vi "LINX I2C Write Test App.vi"() -> ()   [LabVIEW 2011]
uses:
  LVH-LINX.lvlib
panel:
  out "Loop Time":u32
  in  "Stop Button":bool
  in  "Color Box":u32(colorbox)
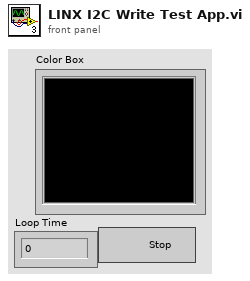
[diagram p1: front panel]
types:
  T1 = typedef "LVH-LINX.lvlib/LINX Ref.ctl" = cluster{"Platform":T2, "Interface":T3, "LINX Device Config":T4}
  T2 = typedef "LVH-LINX.lvlib/Platform.ctl" = enum16{"LINX", "myRIO"}
  T3 = typedef "LVH-LINX.lvlib/Interface.ctl" = enum16{"Serial", "TCP"}
  T4 = typedef "LVH-LINX.lvlib/Device.lvlib/LINX Device Config.ctl" = cluster{"Interface":T3, "COM Port":refnum<visa-resource-name>, "TCP Configuration":T5, "Device Family":T6, "Device ID":u8, "Device Name":string, "TCP Ref":refnum<k5>}
  T5 = typedef "LVH-LINX.lvlib/Device.lvlib/TCP Config.ctl" = cluster{"IP Address":string, "Port":u16}
  T6 = typedef "LVH-LINX.lvlib/Device Family.ctl" = enum8{"National Instruments", "Digilent", "Arduino"}
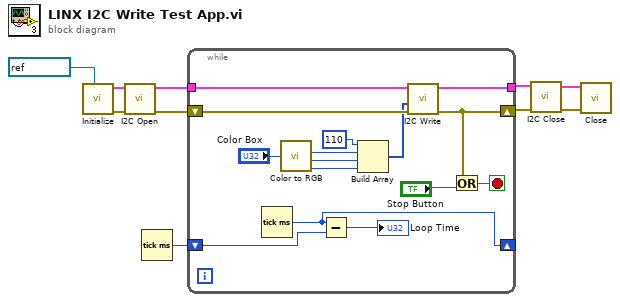
[diagram p0: block diagram]
diagram:
  n1 = call "Initialize.vi"("Serial Port"=refnum<visa-resource-name> "COM5") -> ("Error Out"=w8:errorcluster, "LINX Ref"=w9:T1)  [unwired: 8 in, 1 out]
  n2 = call "I2C Open.vi"("Error In"=w8, "LINX Resource"=w9) -> ("Error Out"=w6:errorcluster, "LINX Resource"=w7:T1)  [unwired: 8 in]
  n3 = Tick Count (ms)() -> (millisecond timer value=w5:u32)
  n4 = while {
    tunnel: [w25] -> w4
    tunnel: w7 -> [w24]
    shift-right: [w16] -> w3
    shift-left: w6 -> [w23]
    shift-right: [w12] -> _
    shift-left: w5 -> [w13]
    stop <- w14 stop-if-true
    n5 = Tick Count (ms)() -> (millisecond timer value=w12:u32)
    n6 = call <vilib>:"Color to RGB.vi"("Color"="Color Box") -> ("R"=w21:u8, "G"=w19:u8, "B"=w18:u8)  [unwired: 1 out]
    n7 = Subtract(x=w12, y=w13) -> (x-y=→"Loop Time":u32)
    n8 = Build Array(u8 110 ("element"), w21, w19, w18) -> (w17:u8[])
    n9 = call "I2C Write.vi"("Error In"=w23, "Data"=w17, "LINX Resource"=w24) -> ("Error Out"=w16:errorcluster, "LINX Resource"=w25:T1)  [unwired: 7 in]
    n10 = Or(x=w16, y="Stop Button") -> (x .or. y?=w14:bool)
  }
  n11 = call "I2C Close.vi"("Error In"=w3, "LINX Resource"=w4) -> ("Error Out"=w2:errorcluster, "LINX Resource"=w1:T1)  [unwired: 8 in]
  n12 = call "Close.vi"("Error In"=w2, "LINX Resource"=w1) -> ()  [unwired: 8 in, 2 out]
